vi "Iterate.vi"(8 "error in (no error)":errorcluster, 11 "Example Actor in":refnum<class "Example Actor.lvclass">) -> (0 "error out":errorcluster, 3 "Example Actor out":refnum<class "Example Actor.lvclass">)   [LabVIEW 2023, in "Example Iterator NR Actor Explicit Iteration.lvlib" / "Example Actor.lvclass"]
doc: "Method called duriong the iterations"
uses:
  Example Actor.lvclass
  Example Actor.lvclass/Example Actor.ctl
  <userlib>/_OpenG.lib/time/time.llb/openg_time.lvlib
  Iterator NR Actor Messages/Notify Iteration Msg/Notify Iteration Msg.lvclass
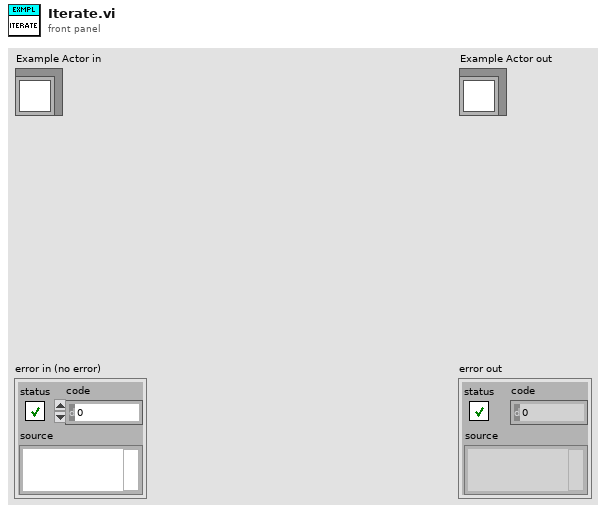
[diagram p1: front panel]
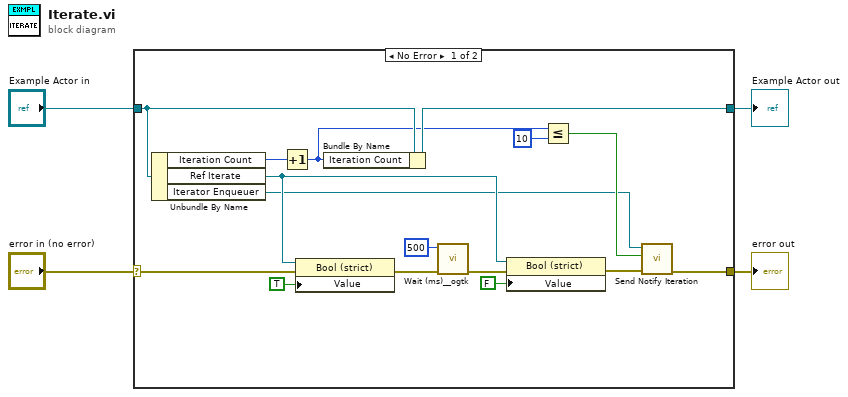
[diagram p0: block diagram]
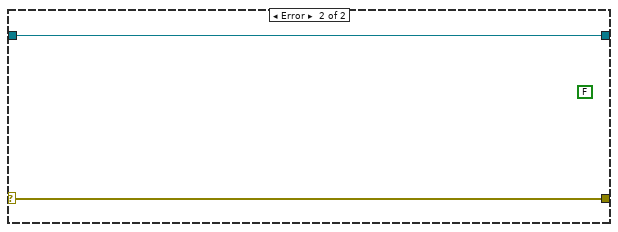
[diagram p2: hidden frame]
diagram:
  n1 = case shown="No Error" "error in (no error)" {
    selector: "error in (no error)" -> [w19 w22]
    tunnel: [w7 w22] -> w3
    tunnel: [w12 w21] -> w1
    tunnel: "Example Actor in" -> [w20 w21]
    frame No Error {
      n2 = Unbundle By Name(w20) -> ("Iteration Count"=w11:i32, "Ref Iterate"=w16:refnum<vi>, "Iterator Enqueuer"=w5:refnum<class "Message Enqueuer.lvclass">)
      n3 = Increment(x=w11) -> (x+1=w10:i32)
      n4 = property class="Bool (strict)"(reference=w16, error in=w19, "Value"=TRUE) -> (error out=w18:errorcluster)  [unwired: 1 out]
      n5 = Bundle By Name(cluster=w20, "Iteration Count"=w10) -> (w12:refnum<class "Example Actor.lvclass">)
      n6 = call <userlib>:"Wait (ms)__ogtk.vi"("error in (no error)"=w18, "milliseconds to wait"=u32 500) -> ("error out"=w17:errorcluster)  [unwired: 8 in, 1 out]
      n7 = property class="Bool (strict)"(reference=w16, error in=w17, "Value"=FALSE) -> (error out=w8:errorcluster)  [unwired: 1 out]
      n8 = Less Or Equal?(x=w10, y=10) -> (x <= y?=w6:bool)
      n9 = call "Send Notify Iteration.vi"("error in (no error)"=w8, "Iterate (T)"=w6, "Message Enqueuer in"=w5) -> ("error out"=w7:errorcluster)  [unwired: 7 in, 1 out]
    }
    frame Error {
      (unwired) FALSE
    }
  }
  "error out" <- w3
  "Example Actor out" <- w1
